vi "Unsubscribe.vi"(8 "error in (no error)":errorcluster, 9 "Subscriber":string, 10 "Topic":string, 11 "Broadcaster in":refnum<class "BroadcastBroker.lvclass">) -> (0 "error out":errorcluster, 3 "Broadcaster out":refnum<class "BroadcastBroker.lvclass">)   [LabVIEW 2015, in "BroadcastBroker.lvclass"]
uses:
  BroadcastBroker.lvclass
  BroadcastBroker.lvclass/BroadcastBroker.ctl
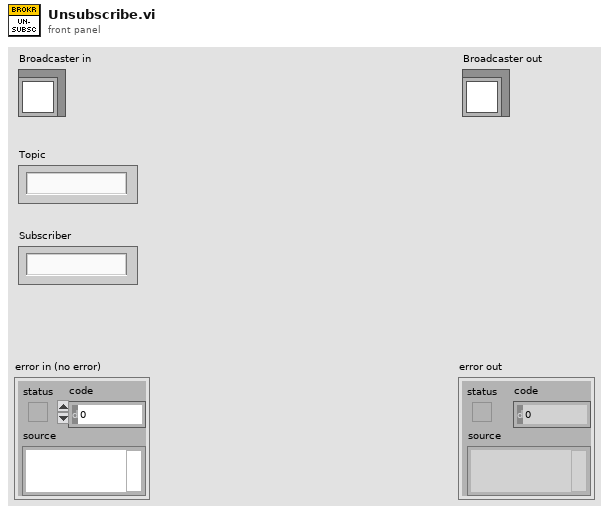
[diagram p1: front panel]
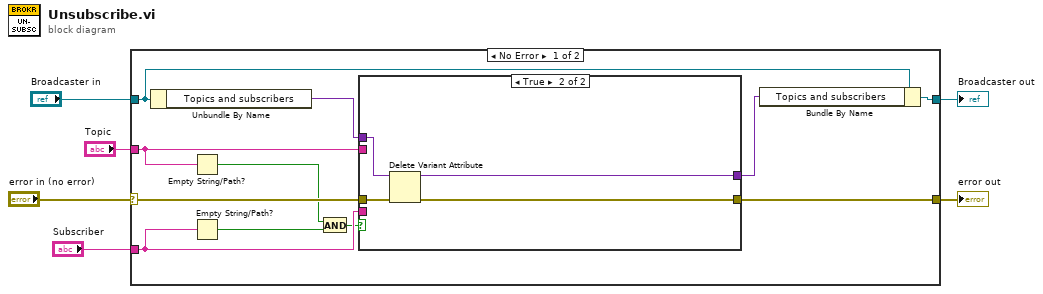
[diagram p0: block diagram]
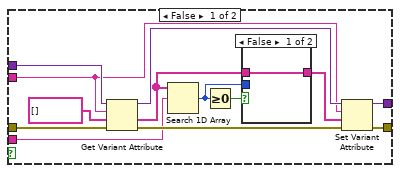
[diagram p2: hidden frame]
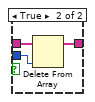
[diagram p3: hidden frame]
diagram:
  n1 = case shown="No Error" "error in (no error)" {
    selector: "error in (no error)" -> [w15 w40]
    tunnel: [w12 w40] -> w5
    tunnel: [w14 w39] -> w3
    tunnel: "Broadcaster in" -> [w17 w39]
    tunnel: "Topic" -> [w11 _]
    tunnel: "Subscriber" -> [w10 _]
    frame No Error {
      n2 = Unbundle By Name(w17) -> ("Topics and subscribers"=w16:variant)
      n3 = Empty String/Path?(string/path=w11) -> (empty?=w8:bool)
      n4 = Empty String/Path?(string/path=w10) -> (empty?=w9:bool)
      n5 = And(x=w8, y=w9) -> (x .and. y?=w7:bool)
      n6 = case shown="True" w7 {
        tunnel: w16 -> [w30 w38]
        tunnel: w15 -> [w29 w37]
        tunnel: [w25 w35] -> w13
        tunnel: [w24 w36] -> w12
        tunnel: w11 -> [w19 _]
        tunnel: w10 -> [w18 _]
        frame False {
          n7 = Get Variant Attribute(Variant=w30, name=w19, default value (empty Variant)=string[] [], error in=w29) -> (duplicate Variant=w26:variant, value=w22:string[], error out=w27:errorcluster)  [unwired: 1 out]
          n8 = Search 1D Array(1D array=w22, element=w18) -> (index of element=w21:i32)  [unwired: 1 in]
          n9 = Greater Or Equal To 0?(x=w21) -> (x >= 0?=w23:bool)
          n10 = case shown="False" w23 {
            tunnel: w22 -> [w31 w34]
            tunnel: w21 -> [_ w33]
            tunnel: [w31 w32] -> w20
            frame False {
            }
            frame True {
              n11 = Delete From Array(array=w34, index=w33) -> (array with subset deleted=w32:string[])  [unwired: 1 in, 1 out]
            }
          }
          n12 = Set Variant Attribute(Variant=w26, name=w19, value=w20, error in=w27) -> (Variant out=w25:variant, error out=w24:errorcluster)  [unwired: 1 out]
        }
        frame True {
          n13 = Delete Variant Attribute(4:w37, 7:w38) -> (0:w36:errorcluster, 3:w35:variant)  [unwired: 1 in, 1 out]
        }
      }
      n14 = Bundle By Name(cluster=w17, "Topics and subscribers"=w13) -> (w14:refnum<class "BroadcastBroker.lvclass">)
    }
    frame Error {
    }
  }
  "error out" <- w5
  "Broadcaster out" <- w3
